vi "Write T.vi"(8 "error in":errorcluster, 10 "T":sgl, 11 "CRDS Cell Data in":refnum<class "CRDS Cell Data.lvclass">) -> (0 "error out":errorcluster, 3 "CRDS Cell Data out":refnum<class "CRDS Cell Data.lvclass">)   [LabVIEW 2014, in "CRDS Lib.lvlib" / "CRDS Cell Data.lvclass"]
doc: "Enter thermistor values for the cell."
uses:
  CRDS Cell Data.lvclass
  CRDS Cell Data.lvclass/CRDS Cell Data.ctl
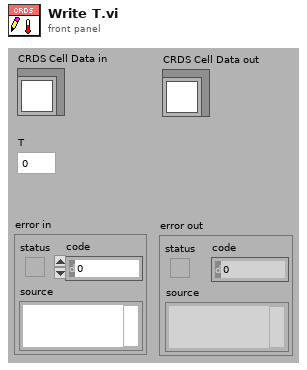
[diagram p1: front panel]
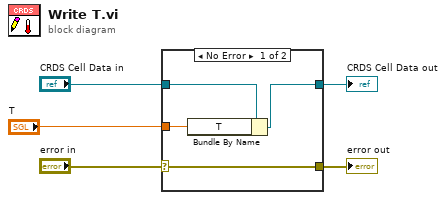
[diagram p0: block diagram]
diagram:
  n1 = case shown="No Error" "error in" {
    selector: "error in" -> [w9 w10]
    tunnel: [w9 w10] -> w4
    tunnel: [w7 w11] -> w2
    tunnel: "CRDS Cell Data in" -> [w8 w11]
    tunnel: "T" -> [w6 _]
    frame No Error {
      n2 = Bundle By Name(cluster=w8, "T"=w6) -> (w7:refnum<class "CRDS Cell Data.lvclass">)
    }
    frame Error {
    }
  }
  "error out" <- w4
  "CRDS Cell Data out" <- w2
